vi "Update Actual Motor Speeds Indicator.vi"(8 "error in (no error)":errorcluster, 9 "value":string, 10 "String":string, 11 "Mode":enum16{"Init", "Idle", "Update"}(ring)) -> (0 "error out":errorcluster, 3 "Actual Motor Speeds":cluster{dbl, dbl}(knob) scale=0.0..1000.0)   [LabVIEW 2023]
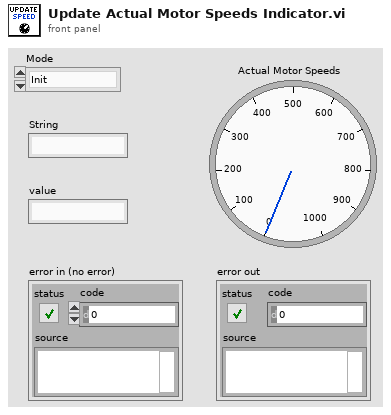
[diagram p1: front panel]
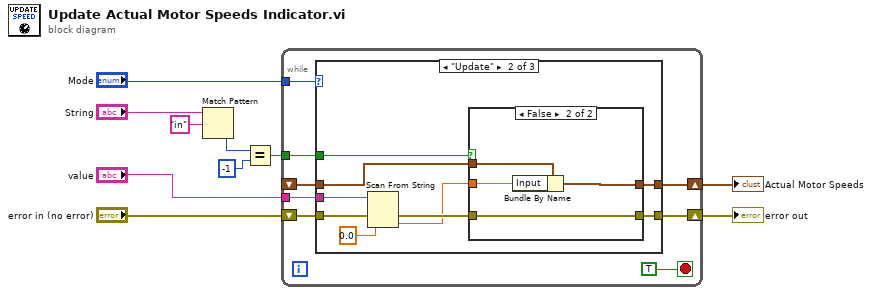
[diagram p0: block diagram]
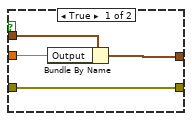
[diagram p3: hidden frame]
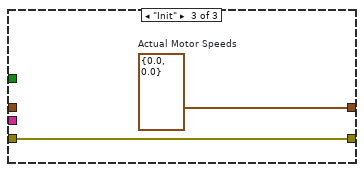
[diagram p4: hidden frame]
diagram:
  n1 = Match Pattern(string="String", regular expression="in") -> (offset past match=w8:i32)  [unwired: 1 in, 3 out]
  n2 = Equal?(x=w8, y=-1) -> (x = y?=w10:bool)
  n3 = while {
    tunnel: w10 -> [w15]
    shift-right: [w18] -> w7
    shift-left: "error in (no error)" -> [w17]
    shift-right: [w16] -> w4
    shift-left: _ -> [w12]
    tunnel: "Mode" -> [w13]
    tunnel: "value" -> [w11]
    stop <- TRUE stop-if-true
    n4 = case shown="\"Update\"" w13 {
      tunnel: [w20 w29 w39] -> w18
      tunnel: w17 -> [w20 w26 w39]
      tunnel: [w19 w28 w38] -> w16
      tunnel: w15 -> [_ w27 _]
      tunnel: w12 -> [w19 w21 _]
      tunnel: w11 -> [_ w22 _]
      frame "Idle", Default {
      }
      frame "Update" {
        n5 = Scan From String(input string=w22, error in=w26, default 1=0.0) -> (error out=w25:errorcluster, output 1=w23:dbl)  [unwired: 2 in, 2 out]
        n6 = case shown="False" w27 {
          tunnel: w25 -> [w33 w37]
          tunnel: [w33 w37] -> w29
          tunnel: w23 -> [w32 w36]
          tunnel: [w31 w35] -> w28
          tunnel: w21 -> [w30 w34]
          frame True {
            n7 = Bundle By Name(cluster=w30, "Output"=w32) -> (w31:cluster{"Input":dbl, "Output":dbl})
          }
          frame False {
            n8 = Bundle By Name(cluster=w34, "Input"=w36) -> (w35:cluster{"Input":dbl, "Output":dbl})
          }
        }
      }
      frame "Init" {
        w38 = cluster{"Input":dbl, "Output":dbl} {"Input"=0.0, "Output"=0.0}  # Actual Motor Speeds
      }
    }
  }
  "Actual Motor Speeds" <- w4
  "error out" <- w7
